vi "Remote Panel Methods Server.vi"() -> ()   [LabVIEW 2023]
doc: "This Server VI serves as a model of how you could allow a client to only run a VI once after connecting and taking control. It starts the remote panel server, polls for a connection, waits until the client runs the VI once, and then locks control and disconnects the client."
panel:
  out "Remote Panel Server Address":string
  out "Remote Panel Server Port":u16
  out "Client Has Control?":bool
  out "Connected Client Address":string
  # "Overview: Demonstrates the use of Remote Panel methods to configure a server for remote panel connections.\nRequirements: LabVIEW Full Development System\nInstructions:\n1. Make sure you have opened this example from Remote Panel Methods.lvproj. The example will not work properly if you open this VI outside of the project.\n2. Navigate to Tools > Options > Web Server and select Enable Remote Panel Server.\n3. Run this VI.\n4. In a different instance of LabVIEW (but the same version of LabVIEW as this instance), run Remote Panel Methods Client.vi and follow the instructions on its front panel."
  # "Server Information"
  # "Client Information"
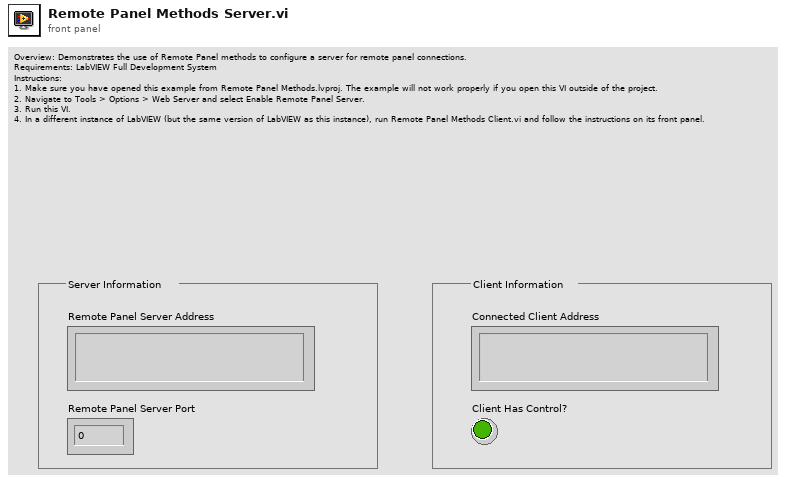
[diagram p1: front panel]
types:
  T1 = enum32{"Bad", "Idle", "Run top level", "Running"}
  T2 = typedef "LVRemotePanelConnectionsTypeDef.ctl" = cluster{"VI Name":string, "Remote":string, "UserName":string, "Port":i32, "Status":enum32{"Viewing", "Waiting For Control", "Controlling"}, "Create Time":timestamp, "Status Time":timestamp, "Control End Time":timestamp}[]
  T3 = cluster{"VI Name":string, "Remote":string, "UserName":string, "Port":i32, "Status":enum32{"Viewing", "Waiting For Control", "Controlling"}, "Create Time":timestamp, "Status Time":timestamp, "Control End Time":timestamp}
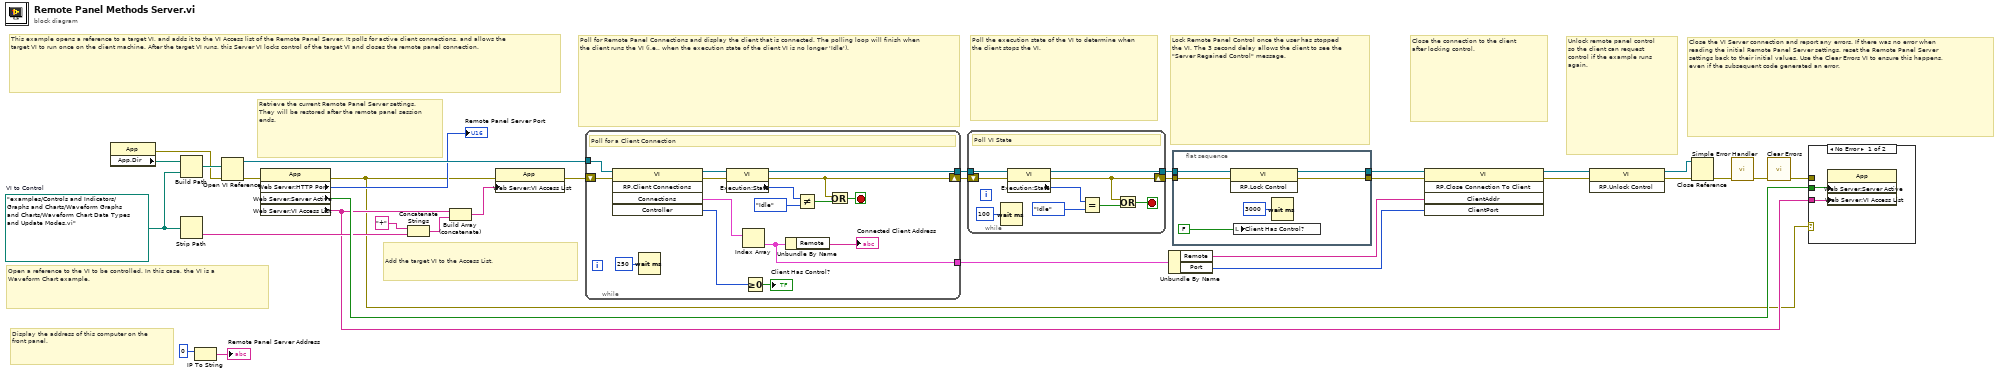
[diagram p0: block diagram]
diagram:
  w8 = path "examples/Controls and Indicators/Graphs and Charts/Waveform Graphs and Charts/Waveform Chart Data Types and Update Modes.vi"  # VI to Control
  # "Display the address of this computer on the front panel."
  # "This example opens a reference to a target VI, and adds it to the VI Access list of the Remote Panel Server. It polls for active client connections, and allows the target VI to run once on the client machine. After the target VI runs, this Server VI locks control of the target VI and closes the remote panel connection."
  # "Retrieve the current Remote Panel Server settings. They will be restored after the remote panel session ends."
  # "Add the target VI to the Access List."
  # "Open a reference to the VI to be controlled. In this case, the VI is a Waveform Chart example."
  # "Close the VI Server connection and report any errors. If there was no error when reading the initial Remote Panel Server settings, reset the Remote Panel Server settings back to their initial values. Use the Clear Errors VI to ensure this happens, even if the subsequent code generated an error."
  # "Unlock remote panel control so the client can request control if the example runs again."
  # "Close the connection to the client after locking control."
  # "Lock Remote Panel Control once the user has stopped the VI. The 3 second delay allows the client to see the \"Server Regained Control\" message."
  # "Poll the execution state of the VI to determine when the client stops the VI."
  # "Poll for Remote Panel Connections and display the client that is connected. The polling loop will finish when the client runs the VI (i.e., when the execution state of the client VI is no longer 'Idle')."
  n1 = property class="App"() -> (error out=w9:errorcluster, "App.Dir"=w10:path)  [unwired: 2 in, 1 out]
  n2 = Build Path(base path=w10, name or relative path=w8) -> (appended path=w11:path)
  n3 = Strip Path(path=w8) -> (name=w15:string)  [unwired: 1 out]
  n4 = IP To String(2:u32 0 ("net address")) -> (0:→"Remote Panel Server Address":string)  [unwired: 1 in]
  n5 = Open VI Reference(vi path=w11, error in (no error)=w9) -> (vi reference=w29:refnum<vi>, error out=w28:errorcluster)  [unwired: 4 in]
  n6 = property class="App"(error in=w28) -> (error out=w4:errorcluster, "Web Server:HTTP Port"=→"Remote Panel Server Port":u16, "Web Server:Server Active"=w16:bool, "Web Server:VI Access List"=w13:string[])  [unwired: 1 in, 1 out]
  n7 = Concatenate Strings("+" ("string"), w15) -> (w14:string)
  n8 = Build Array (concatenate)(w13, w14) -> (w12:string[])
  n9 = property class="App"(error in=w4, "Web Server:VI Access List"=w12) -> (error out=w19:errorcluster)  [unwired: 1 in, 1 out]
  n10 = while {
    tunnel: w29 -> [w46]
    tunnel: [w38] -> w26
    shift-right: [w36] -> w27
    shift-left: w19 -> [w45]
    tunnel: [w34] -> w3
    stop <- w47 stop-if-true
    # "Poll for a Client Connection"
    n11 = invoke class="VI" method="RP.Client Connections"(reference=w46, error in=w45) -> (reference out=w39:refnum<vi>, error out=w41:errorcluster, "Connections"=w48:T2, "Controller"=w37:i32)  [unwired: 3 in, 1 out]
    n12 = Wait (ms)(milliseconds to wait=u32 250) -> ()  [unwired: 1 out]
    n13 = property class="VI"(reference=w39, error in=w41) -> (reference out=w38:refnum<vi>, error out=w36:errorcluster, "Execution:State"=w43:T1)
    n14 = Index Array(array=w48) -> (element=w34:T3)  [unwired: 1 in]
    n15 = Greater Or Equal To 0?(x=w37) -> (x >= 0?=→"Client Has Control?":bool)
    n16 = Unbundle By Name(w34) -> ("Remote"=→"Connected Client Address":string)
    n17 = Not Equal?(x=w43, y=T1."Idle" ("Execution:State")) -> (x != y?=w40:bool)
    n18 = Or(x=w36, y=w40) -> (x .or. y?=w47:bool)
  }
  n19 = while {
    tunnel: w26 -> [w56]
    tunnel: [w51] -> w22
    shift-right: [w50] -> w25
    shift-left: w27 -> [w58]
    stop <- w53 stop-if-true
    # "Poll VI State"
    n20 = Wait (ms)(milliseconds to wait=u32 100) -> ()  [unwired: 1 out]
    n21 = property class="VI"(reference=w56, error in=w58) -> (reference out=w51:refnum<vi>, error out=w50:errorcluster, "Execution:State"=w55:T1)
    n22 = Equal?(x=w55, y=T1."Idle" ("Execution:State")) -> (x = y?=w52:bool)
    n23 = Or(x=w50, y=w52) -> (x .or. y?=w53:bool)
  }
  n24 = Unbundle By Name(w3) -> ("Remote"=w21:string, "Port"=w20:i32)
  n25 = flat-sequence {
    tunnel: w25 -> [w64]
    tunnel: [w63] -> w24
    tunnel: [w62] -> w23
    tunnel: w22 -> [w61]
    frame #0 {
      n26 = invoke class="VI" method="RP.Lock Control"(reference=w61, error in=w64) -> (reference out=w62:refnum<vi>, error out=w63:errorcluster)  [unwired: 1 in, 1 out]
      n27 = local write "Client Has Control?"(FALSE ("Client Has Control?")) -> ()
      n28 = Wait (ms)(milliseconds to wait=u32 3000) -> ()  [unwired: 1 out]
    }
  }
  n29 = invoke class="VI" method="RP.Close Connection To Client"(reference=w23, error in=w24, "ClientAddr"=w21, "ClientPort"=w20) -> (reference out=w32:refnum<vi>, error out=w33:errorcluster)  [unwired: 1 in, 3 out]
  n30 = invoke class="VI" method="RP.Unlock Control"(reference=w32, error in=w33) -> (reference out=w31:refnum<vi>, error out=w30:errorcluster)  [unwired: 1 in, 1 out]
  n31 = Close Reference(reference=w31, error in (no error)=w30) -> (error out=w17:errorcluster)
  n32 = call <vilib>:"Simple Error Handler.vi"("error in (no error)"=w17) -> ("error out"=w6:errorcluster)  [unwired: 4 in, 4 out]
  n33 = call <vilib>:"Clear Errors.vi"("error in (no error)"=w6) -> ("error out"=w5:errorcluster)  [unwired: 5 in, 1 out]
  n34 = case shown="No Error" w4 {
    tunnel: w16 -> [w66 _]
    tunnel: w13 -> [w65 _]
    tunnel: w5 -> [_ _]
    frame No Error {
      n35 = property class="App"("Web Server:Server Active"=w66, "Web Server:VI Access List"=w65) -> ()  [unwired: 2 in, 2 out]
    }
    frame Error {
    }
  }
